vi "MotorTrapezoidalMotion.vi"(8 "error in":errorcluster, 9 "Desired Power":dbl, 10 "Motor Power Step":dbl) -> (0 "error out":errorcluster, 2 "Motor Power":dbl)   [LabVIEW 2018]
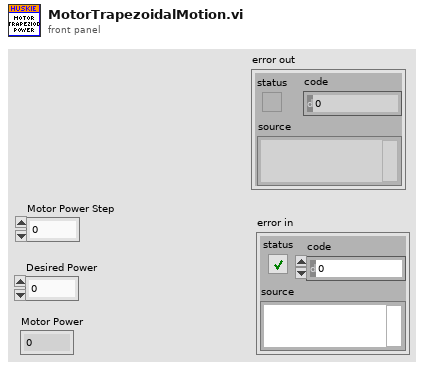
[diagram p1: front panel]
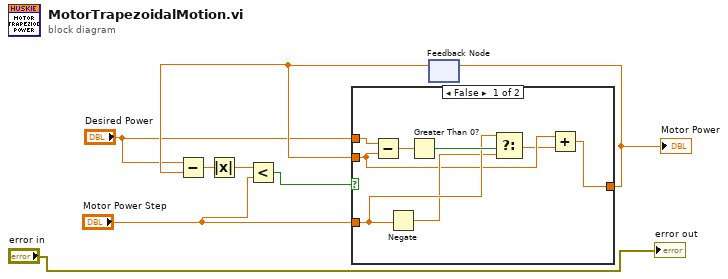
[diagram p0: block diagram]
diagram:
  n1 = feedback #1() -> (w7:dbl)  [unwired: 1 in]
  n2 = Subtract(x="Desired Power", y=w7) -> (x-y=w6:dbl)
  n3 = Absolute Value(x=w6) -> (abs(x)=w5:dbl)
  n4 = Less?(x=w5, y="Motor Power Step") -> (x < y?=w3:bool)
  n5 = case shown="False" w3 {
    tunnel: "Motor Power Step" -> [w12 _]
    tunnel: w7 -> [w10 _]
    tunnel: [w16 w17] -> w8
    tunnel: "Desired Power" -> [w15 w17]
    frame False {
      n6 = Subtract(x=w15, y=w10) -> (x-y=w14:dbl)
      n7 = Negate(x=w12) -> (-x=w11:dbl)
      n8 = Greater Than 0?(x=w14) -> (x > 0?=w13:bool)
      n9 = Select(t=w12, s=w13, f=w11) -> (s? t:f=w9:dbl)
      n10 = Add(x=w10, y=w9) -> (x+y=w16:dbl)
    }
    frame True {
    }
  }
  "Motor Power" <- w8
  n11 = feedback-in #1(w8) -> ()
  "error out" <- "error in"
